vi "HEWH Power Cluster Calcs.vi"(0 "MW100 Data Cluster":T2, 5 "Data (Label, Channel, Data)":string[][](array[string]), 11 "Error In":errorcluster, 12 "LV Program":T1) -> (3 "PowerData":T3, 4 "MW100 Data Cluster Output":T2, 6 "Tank Display":dbl[](array[numeric]), 15 "Error Out":errorcluster)   [LabVIEW 2016]
uses:
  Type Definitions/HEWH Power Data.ctl
  Type Definitions/HEWH MW100 Data Cluster.ctl
  Utility/Save File/File Setup (Public)/Type Definition/Save File DOE LabView Program.ctl
  <vilib>/Analysis/NI_AALBase.lvlib
  Utility/Save File/File Setup.lvlib
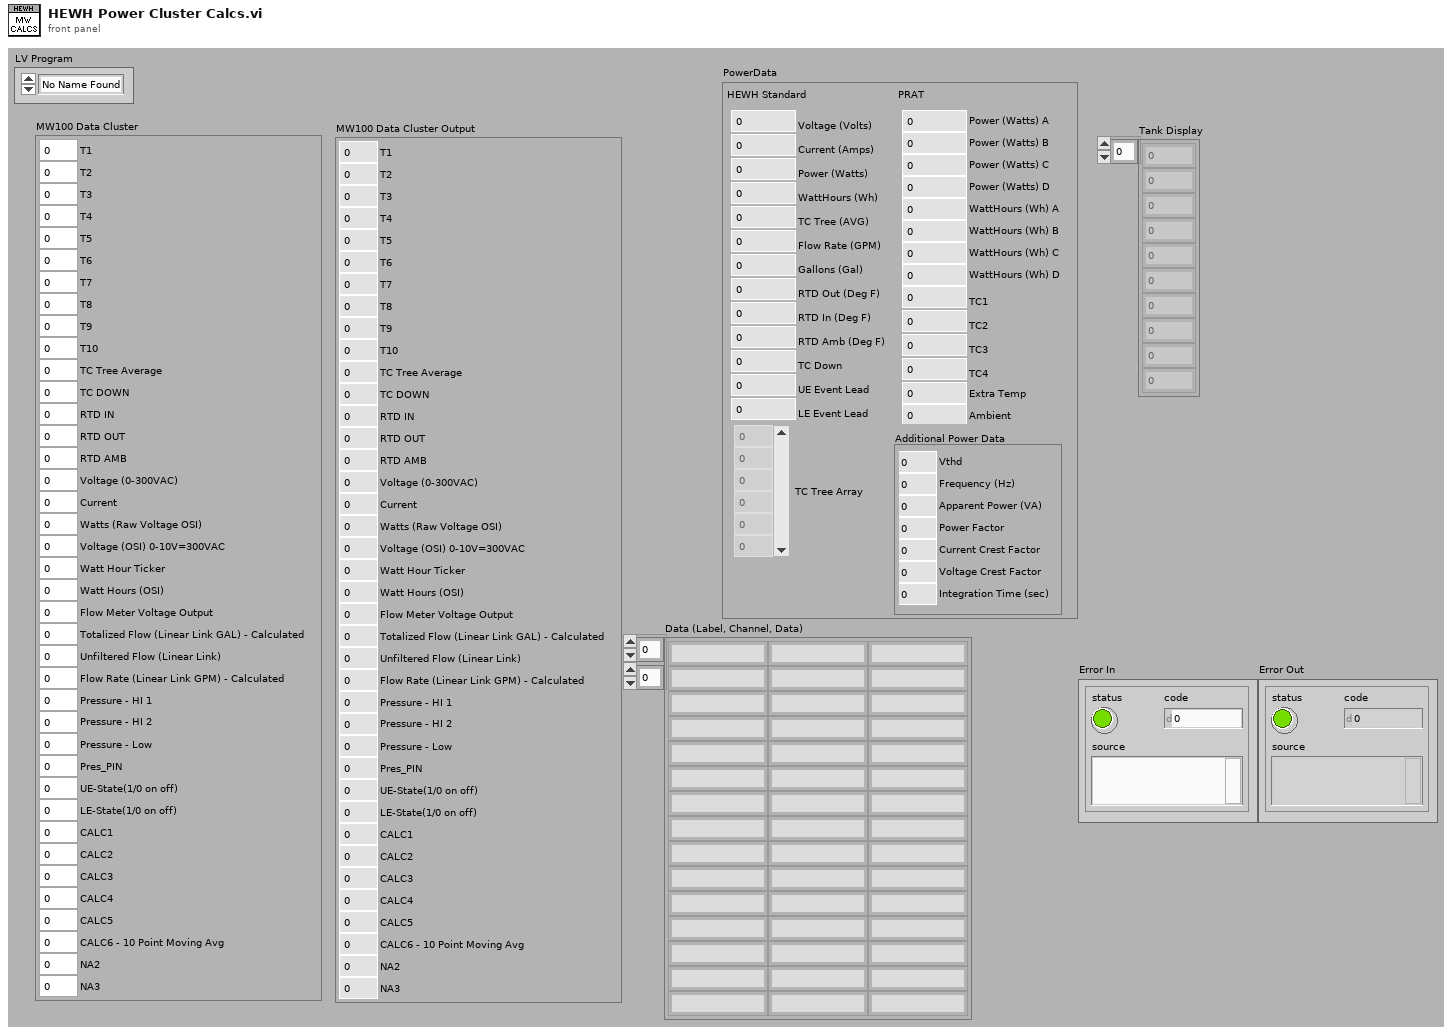
[diagram p1: front panel]
types:
  T1 = typedef "File Setup.lvlib/Save File DOE LabView Program.ctl" = enum16{"No Name Found", "DOE Stand", "Dishwasher Kitchen", "Portable Stand", "HEWH", "Dryer", "Dryer WILT", "HCC", "PRAT", "HEWH RLT", "Refrigeration"}
  T2 = typedef "HEWH MW100 Data Cluster.ctl" = cluster{"T1":dbl, "T2":dbl, "T3":dbl, "T4":dbl, "T5":dbl, "T6":dbl, "T7":dbl, "T8":dbl, "T9":dbl, "T10":dbl, "TC Tree Average":dbl, "TC DOWN":dbl, "RTD IN":dbl, "RTD OUT":dbl, "RTD AMB":dbl, "Voltage (0-300VAC)":dbl, "Current":dbl, "Watts (Raw Voltage OSI)":dbl, "Voltage (OSI) 0-10V=300VAC":dbl, "Watt Hour Ticker":dbl, "Watt Hours (OSI)":dbl, "Flow Meter Voltage Output":dbl, "Totalized Flow (Linear Link GAL) - Calculated":dbl, "Unfiltered Flow (Linear Link)":dbl, "Flow Rate (Linear Link GPM) - Calculated":dbl, "Pressure - HI 1":dbl, "Pressure - HI 2":dbl, "Pressure - Low":dbl, "Pres_PIN":dbl, "UE-State(1/0 on off)":dbl, "LE-State(1/0 on off)":dbl, "CALC1":dbl, "CALC2":dbl, "CALC3":dbl, "CALC4":dbl, "CALC5":dbl, "CALC6 - 10 Point Moving Avg":dbl, "NA2":dbl, "NA3":dbl}
  T3 = typedef "HEWH Power Data.ctl" = cluster{"HEWH Standard":cluster{"Voltage (Volts)":dbl, "Current (Amps)":dbl, "Power (Watts)":dbl, "WattHours (Wh)":dbl, "TC Tree (AVG)":dbl, "Flow Rate (GPM)":dbl, "Gallons (Gal)":dbl, "RTD Out (Deg F)":dbl, "RTD In (Deg F)":dbl, "RTD Amb (Deg F)":dbl, "TC Down":dbl, "UE Event Lead":i32, "LE Event Lead":i32, "TC Tree Array":dbl[]}, "PRAT":cluster{"Power (Watts) A":dbl, "Power (Watts) B":dbl, "Power (Watts) C":dbl, "Power (Watts) D":dbl, "TC1":dbl, "TC2":dbl, "TC3":dbl, "TC4":dbl, "WattHours (Wh) A":dbl, "WattHours (Wh) B":dbl, "WattHours (Wh) C":dbl, "WattHours (Wh) D":dbl, "Ambient":dbl, "Extra Temp":dbl}, "Additional Power Data":cluster{"Vthd":dbl, "Frequency (Hz)":dbl, "Apparent Power (VA)":dbl, "Power Factor":dbl, "Current Crest Factor":dbl, "Voltage Crest Factor":dbl, "Integration Time (sec)":dbl}}
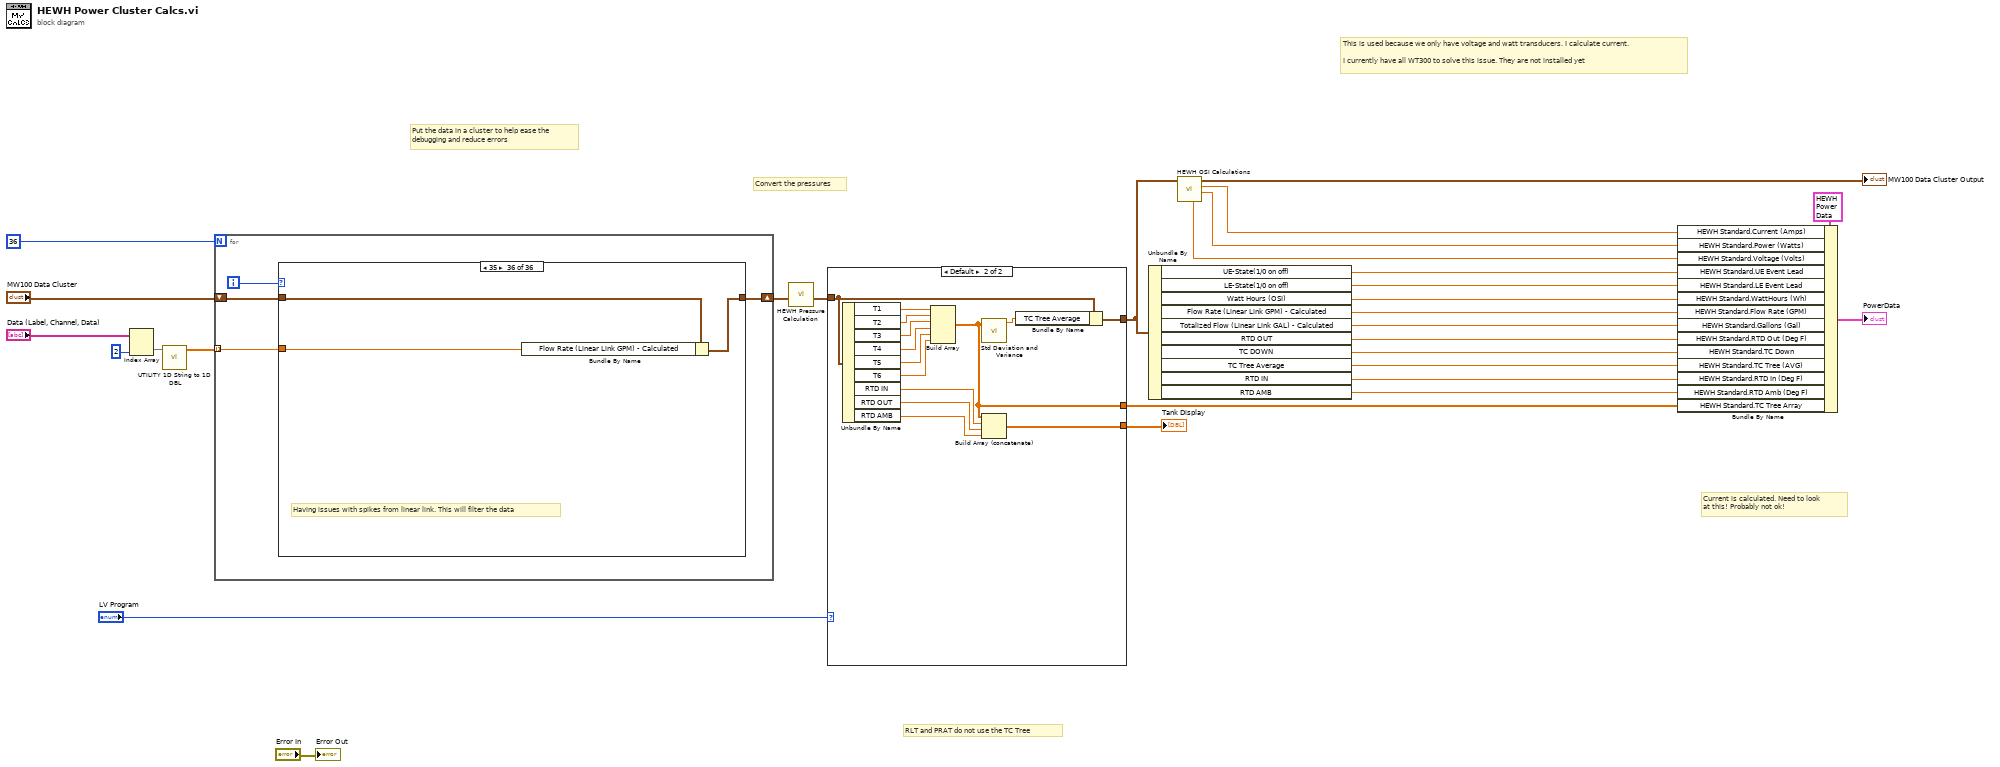
[diagram p0: block diagram]
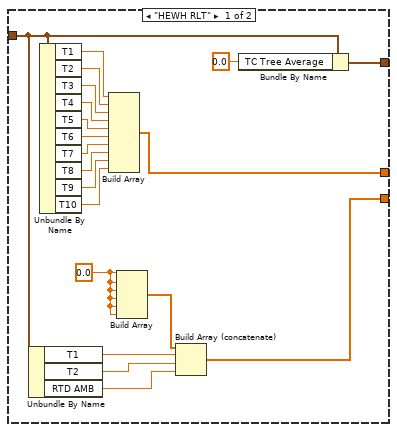
[diagram p2: hidden frame]
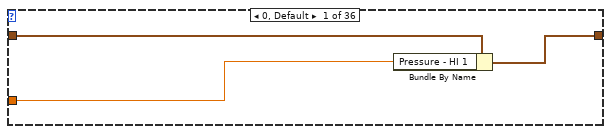
[diagram p3: hidden frame]
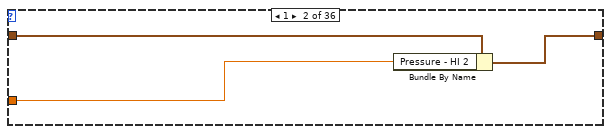
[diagram p4: hidden frame]
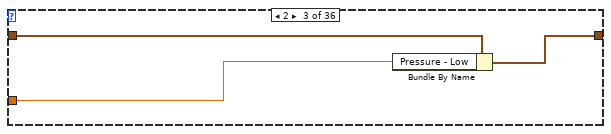
[diagram p5: hidden frame]
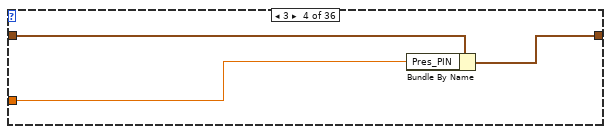
[diagram p6: hidden frame]
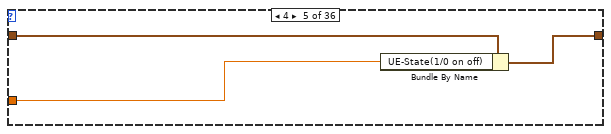
[diagram p7: hidden frame]
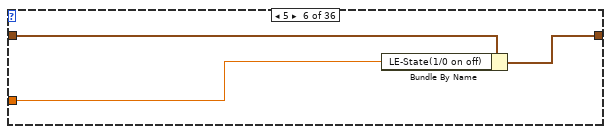
[diagram p8: hidden frame]
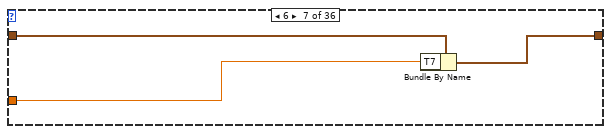
[diagram p9: hidden frame]
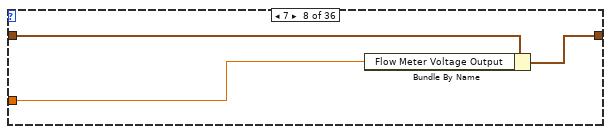
[diagram p10: hidden frame]
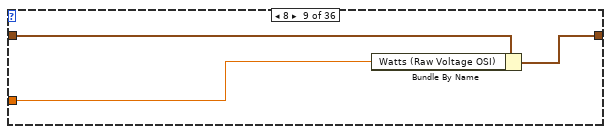
[diagram p11: hidden frame]
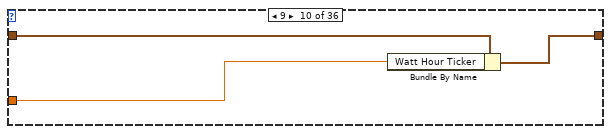
[diagram p12: hidden frame]
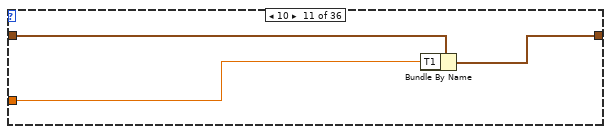
[diagram p13: hidden frame]
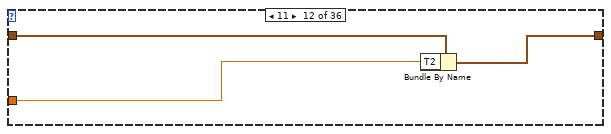
[diagram p14: hidden frame]
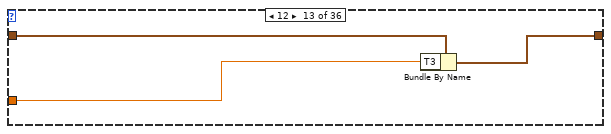
[diagram p15: hidden frame]
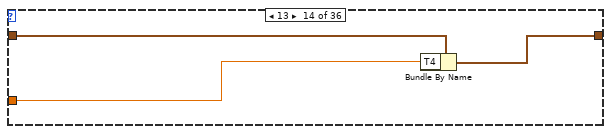
[diagram p16: hidden frame]
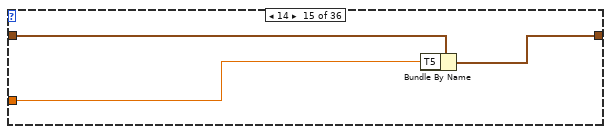
[diagram p17: hidden frame]
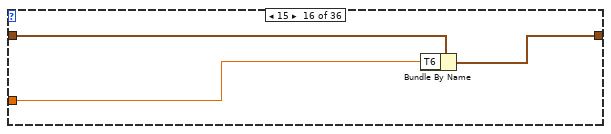
[diagram p18: hidden frame]
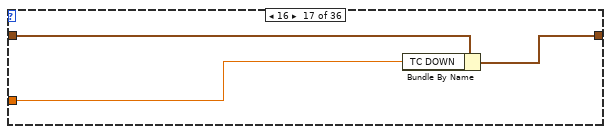
[diagram p19: hidden frame]
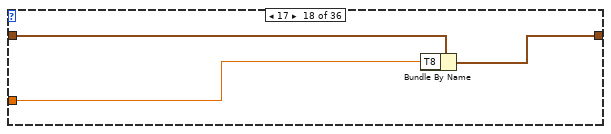
[diagram p20: hidden frame]
diagram:
  # "RLT and PRAT do not use the TC Tree"
  # "Convert the pressures"
  # "Put the data in a cluster to help ease the\ndebugging and reduce errors"
  # "This is used because we only have voltage and watt transducers. I calculate current.\n\nI currently have all WT300 to solve this issue. They are not installed yet"
  # "Current is calculated. Need to look\nat this! Probably not ok!"
  n1 = Index Array(array="Data (Label, Channel, Data)", index (col)=2 ("disabled index (col)")) -> (element=w13:string[])  [unwired: 1 in]
  n2 = call "UTILITY 1D String to 1D DBL.vi"("Save Data"=w13) -> ("DBL"=w14:dbl[])  [unwired: 10 in]
  n3 = for {
    N: 36 -> [_]
    tunnel: w14 -> [w31] mode=indexing
    shift-right: [w30] -> w15
    shift-left: "MW100 Data Cluster" -> [w32]
    i -> [w33]
    n4 = case shown="35" w33 {
      tunnel: w32 -> [w36 w39 w42 w45 w48 w51 w54 w57 w60 w63 w66 w69 w72 w75 w78 w81 w84 w87 w90 w93 w96 w99 w102 w105 w108 w111 w114 w117 w120 w123 w126 w129 w132 w135 w138 w141]
      tunnel: [w35 w38 w41 w44 w47 w50 w53 w56 w59 w62 w65 w68 w71 w74 w77 w80 w83 w86 w89 w92 w95 w98 w101 w104 w107 w110 w113 w116 w119 w122 w125 w128 w131 w134 w137 w140] -> w30
      tunnel: w31 -> [w34 w37 w40 w43 w46 w49 w52 w55 w58 w61 w64 w67 w70 w73 w76 w79 w82 w85 w88 w91 w94 w97 w100 w103 w106 w109 w112 w115 w118 w121 w124 w127 w130 w133 w136 w139]
      frame 0, Default {
        n5 = Bundle By Name(cluster=w36, "Pressure - HI 1"=w34) -> (w35:T2)
      }
      frame 1 {
        n6 = Bundle By Name(cluster=w39, "Pressure - HI 2"=w37) -> (w38:T2)
      }
      frame 2 {
        n7 = Bundle By Name(cluster=w42, "Pressure - Low"=w40) -> (w41:T2)
      }
      frame 3 {
        n8 = Bundle By Name(cluster=w45, "Pres_PIN"=w43) -> (w44:T2)
      }
      frame 4 {
        n9 = Bundle By Name(cluster=w48, "UE-State(1/0 on off)"=w46) -> (w47:T2)
      }
      frame 5 {
        n10 = Bundle By Name(cluster=w51, "LE-State(1/0 on off)"=w49) -> (w50:T2)
      }
      frame 6 {
        n11 = Bundle By Name(cluster=w54, "T7"=w52) -> (w53:T2)
      }
      frame 7 {
        n12 = Bundle By Name(cluster=w57, "Flow Meter Voltage Output"=w55) -> (w56:T2)
      }
      frame 8 {
        n13 = Bundle By Name(cluster=w60, "Watts (Raw Voltage OSI)"=w58) -> (w59:T2)
      }
      frame 9 {
        n14 = Bundle By Name(cluster=w63, "Watt Hour Ticker"=w61) -> (w62:T2)
      }
      frame 10 {
        n15 = Bundle By Name(cluster=w66, "T1"=w64) -> (w65:T2)
      }
      frame 11 {
        n16 = Bundle By Name(cluster=w69, "T2"=w67) -> (w68:T2)
      }
      frame 12 {
        n17 = Bundle By Name(cluster=w72, "T3"=w70) -> (w71:T2)
      }
      frame 13 {
        n18 = Bundle By Name(cluster=w75, "T4"=w73) -> (w74:T2)
      }
      frame 14 {
        n19 = Bundle By Name(cluster=w78, "T5"=w76) -> (w77:T2)
      }
      frame 15 {
        n20 = Bundle By Name(cluster=w81, "T6"=w79) -> (w80:T2)
      }
      frame 16 {
        n21 = Bundle By Name(cluster=w84, "TC DOWN"=w82) -> (w83:T2)
      }
      frame 17 {
        n22 = Bundle By Name(cluster=w87, "T8"=w85) -> (w86:T2)
      }
      frame 18 {
        n23 = Bundle By Name(cluster=w90, "T9"=w88) -> (w89:T2)
      }
      frame 19 {
        n24 = Bundle By Name(cluster=w93, "T10"=w91) -> (w92:T2)
      }
      frame 20 {
        n25 = Bundle By Name(cluster=w96, "RTD IN"=w94) -> (w95:T2)
      }
      frame 21 {
        n26 = Bundle By Name(cluster=w99, "RTD OUT"=w97) -> (w98:T2)
      }
      frame 22 {
        n27 = Bundle By Name(cluster=w102, "RTD AMB"=w100) -> (w101:T2)
      }
      frame 23 {
        n28 = Bundle By Name(cluster=w105, "Voltage (OSI) 0-10V=300VAC"=w103) -> (w104:T2)
      }
      frame 24 {
        n29 = Bundle By Name(cluster=w108, "NA2"=w106) -> (w107:T2)
      }
      frame 25 {
        n30 = Bundle By Name(cluster=w111, "NA3"=w109) -> (w110:T2)
      }
      frame 26 {
        n31 = Bundle By Name(cluster=w114, "CALC1"=w112) -> (w113:T2)
      }
      frame 27 {
        n32 = Bundle By Name(cluster=w117, "Watt Hours (OSI)"=w115) -> (w116:T2)
      }
      frame 28 {
        n33 = Bundle By Name(cluster=w120, "CALC2"=w118) -> (w119:T2)
      }
      frame 29 {
        n34 = Bundle By Name(cluster=w123, "CALC3"=w121) -> (w122:T2)
      }
      frame 30 {
        n35 = Bundle By Name(cluster=w126, "Unfiltered Flow (Linear Link)"=w124) -> (w125:T2)
      }
      frame 31 {
        n36 = Bundle By Name(cluster=w129, "CALC4"=w127) -> (w128:T2)
      }
      frame 32 {
        n37 = Bundle By Name(cluster=w132, "CALC5"=w130) -> (w131:T2)
      }
      frame 33 {
        n38 = Bundle By Name(cluster=w135, "Totalized Flow (Linear Link GAL) - Calculated"=w133) -> (w134:T2)
      }
      frame 34 {
        n39 = Bundle By Name(cluster=w138, "CALC6 - 10 Point Moving Avg"=w136) -> (w137:T2)
      }
      frame 35 {
        # "Having issues with spikes from linear link. This will filter the data"
        n40 = Bundle By Name(cluster=w141, "Flow Rate (Linear Link GPM) - Calculated"=w139) -> (w140:T2)
      }
    }
  }
  n41 = call "HEWH Pressure Calculation.vi"("MW100 Data Cluster"=w15) -> ("Pressure Adjusted"=w16:T2)  [unwired: 10 in]
  n42 = case shown="Default" "LV Program" {
    tunnel: w16 -> [w148 w174]
    tunnel: [w150 w167] -> w2
    tunnel: [w151 w166] -> w3
    tunnel: [w142 w162] -> w9
    frame "HEWH RLT" {
      w147 = 0.0
      n43 = Unbundle By Name(w148) -> ("T1"=w145:dbl, "T2"=w144:dbl, "RTD AMB"=w143:dbl)
      n44 = Unbundle By Name(w148) -> ("T1"=w156:dbl, "T2"=w157:dbl, "T3"=w158:dbl, "T4"=w159:dbl, "T5"=w160:dbl, "T6"=w161:dbl, "T7"=w155:dbl, "T8"=w154:dbl, "T9"=w153:dbl, "T10"=w152:dbl)
      n45 = Build Array(w156, w157, w158, w159, w160, w161, w155, w154, w153, w152) -> (w151:dbl[])
      n46 = Build Array(w147, w147, w147, w147, w147, w147) -> (w146:dbl[])
      n47 = Build Array (concatenate)(w146, w145, w144, w143) -> (w142:dbl[])
      n48 = Bundle By Name(cluster=w148, "TC Tree Average"=0.0) -> (w150:T2)
    }
    frame Default {
      n49 = Unbundle By Name(w174) -> ("T1"=w168:dbl, "T2"=w169:dbl, "T3"=w170:dbl, "T4"=w171:dbl, "T5"=w172:dbl, "T6"=w173:dbl, "RTD IN"=w165:dbl, "RTD OUT"=w164:dbl, "RTD AMB"=w163:dbl)
      n50 = Build Array(w168, w169, w170, w171, w172, w173) -> (w166:dbl[])
      n51 = call <vilib>:"Std Deviation and Variance.vi"("X"=w166) -> ("mean"=w175:dbl)  [unwired: 1 in, 2 out]
      n52 = Build Array (concatenate)(w166, w165, w164, w163) -> (w162:dbl[])
      n53 = Bundle By Name(cluster=w174, "TC Tree Average"=w175) -> (w167:T2)
    }
  }
  "Tank Display" <- w9
  n54 = Unbundle By Name(w2) -> ("UE-State(1/0 on off)"=w20:dbl, "LE-State(1/0 on off)"=w19:dbl, "Watt Hours (OSI)"=w22:dbl, "Flow Rate (Linear Link GPM) - Calculated"=w23:dbl, "Totalized Flow (Linear Link GAL) - Calculated"=w24:dbl, "RTD OUT"=w25:dbl, "TC DOWN"=w26:dbl, "TC Tree Average"=w27:dbl, "RTD IN"=w18:dbl, "RTD AMB"=w17:dbl)
  n55 = call "HEWH OSI Calculations.vi"("Pressure Adjusted in"=w2) -> ("Power (Watts)"=w6:dbl, "Current (Amps)"=w7:dbl, "Pressure Adjusted out"=→"MW100 Data Cluster Output":T2, "Voltage (Volts)"=w5:dbl)  [unwired: 6 in, 1 out]
  n56 = Bundle By Name(cluster=T3 {"HEWH Standard"={"Voltage (Volts)"=-1.0, "Current (Amps)"=-1.0, "Power (Watts)"=-1.0, "WattHours (Wh)"=-1.0, "TC Tree (AVG)"=0.0, "Flow Rate (GPM)"=0.0, "Gallons (Gal)"=0.0, "RTD Out (Deg F)"=0.0, "RTD In (Deg F)"=0.0, "RTD Amb (Deg F)"=0.0, "TC Down"=0.0, "UE Event Lead"=0, "LE Event Lead"=0, "TC Tree Array"=[]}, "PRAT"={"Power (Watts) A"=4192.0, "Power (Watts) B"=4192.0, "Power (Watts) C"=4192.0, "Power (Watts) D"=4192.0, "TC1"=0.0, "TC2"=0.0, "TC3"=0.0, "TC4"=0.0, "WattHours (Wh) A"=4192.0, "WattHours (Wh) B"=4192.0, "WattHours (Wh) C"=4192.0, "WattHours (Wh) D"=4192.0, "Ambient"=0.0, "Extra Temp"=0.0}, "Additional Power Data"={"Vthd"=236.2, "Frequency (Hz)"=236.2, "Apparent Power (VA)"=236.2, "Power Factor"=236.2, "Current Crest Factor"=236.2, "Voltage Crest Factor"=236.2, "Integration Time (sec)"=236.2}} ("PowerData"), "HEWH Standard.Current (Amps)"=w7, "HEWH Standard.Power (Watts)"=w6, "HEWH Standard.Voltage (Volts)"=w5, "HEWH Standard.UE Event Lead"=w20, "HEWH Standard.LE Event Lead"=w19, "HEWH Standard.WattHours (Wh)"=w22, "HEWH Standard.Flow Rate (GPM)"=w23, "HEWH Standard.Gallons (Gal)"=w24, "HEWH Standard.RTD Out (Deg F)"=w25, "HEWH Standard.TC Down"=w26, "HEWH Standard.TC Tree (AVG)"=w27, "HEWH Standard.RTD In (Deg F)"=w18, "HEWH Standard.RTD Amb (Deg F)"=w17, "HEWH Standard.TC Tree Array"=w3) -> (→"PowerData":T3)
  "Error Out" <- "Error In"
